vi "arraytest.vi"() -> ()   [LabVIEW 2010]
panel:
  out "Array 4":i32[][](array[numeric])
  out "Array 3":i32[](array[numeric])
  out "Array 2":bool[](array[boolean])
  out "Array":bool[][](array[boolean])
  out "x+y 2":dbl
  in  "Stopp 2":bool
  out "zeit":dbl
  out "Teil-Array":dbl[](array[numeric])
  in  "Index (Zeile)":i32
  in  "Zykluslänge [s]":i32
  out "XY-Graph":cluster{dbl[], dbl[]}[](graph)
  out "Boolesch 2":bool=TRUE
  out "Boolesch":bool=TRUE
  in  "Stopp":bool
  out "x+y":dbl[](array[numeric])
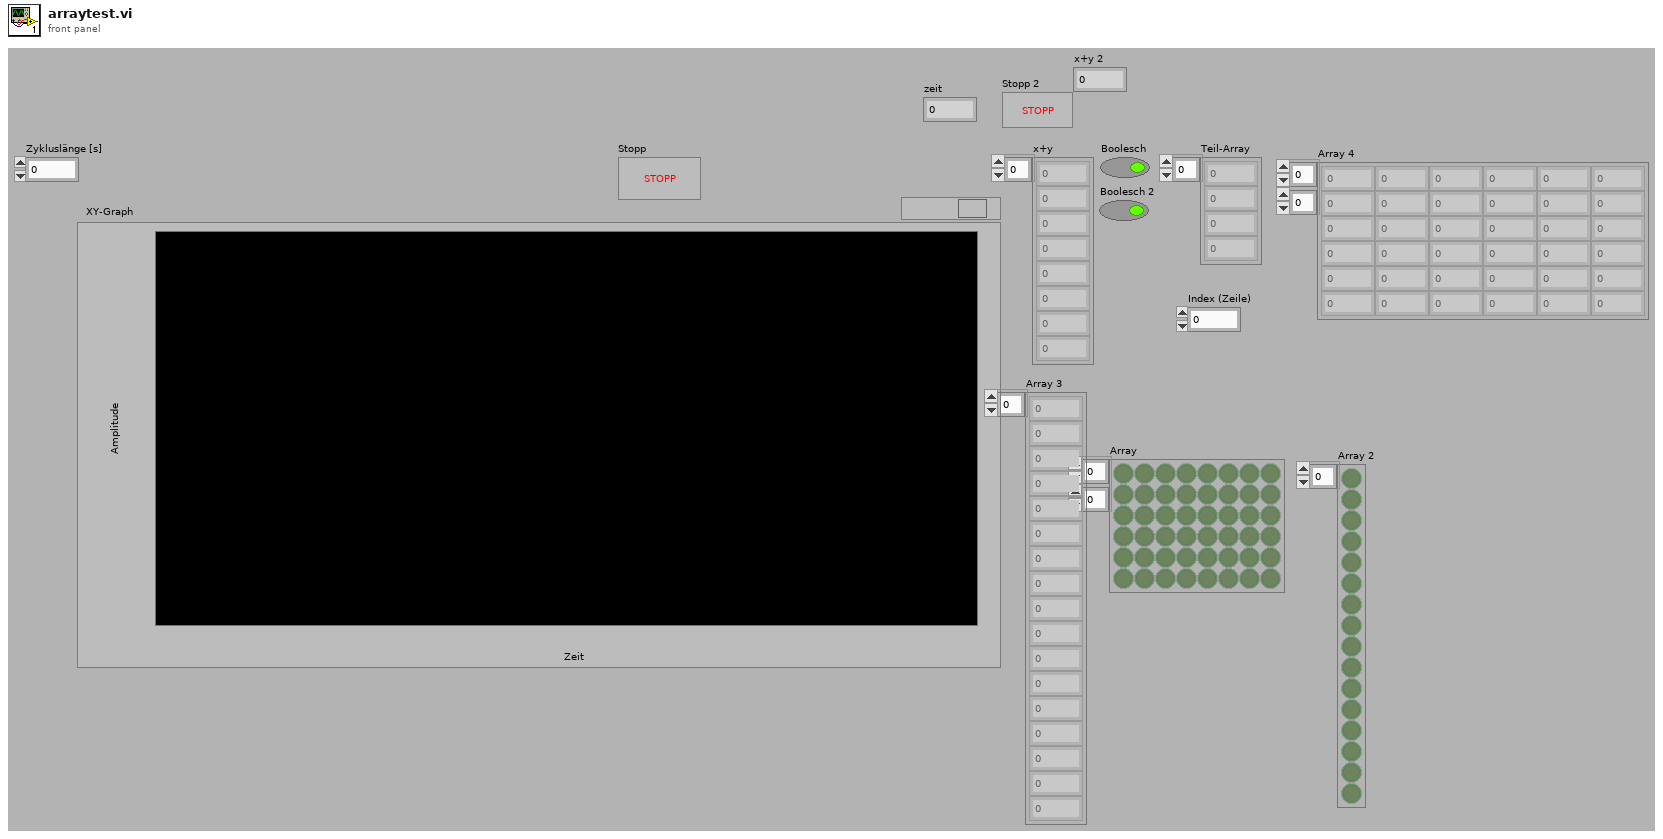
[diagram p1: front panel]
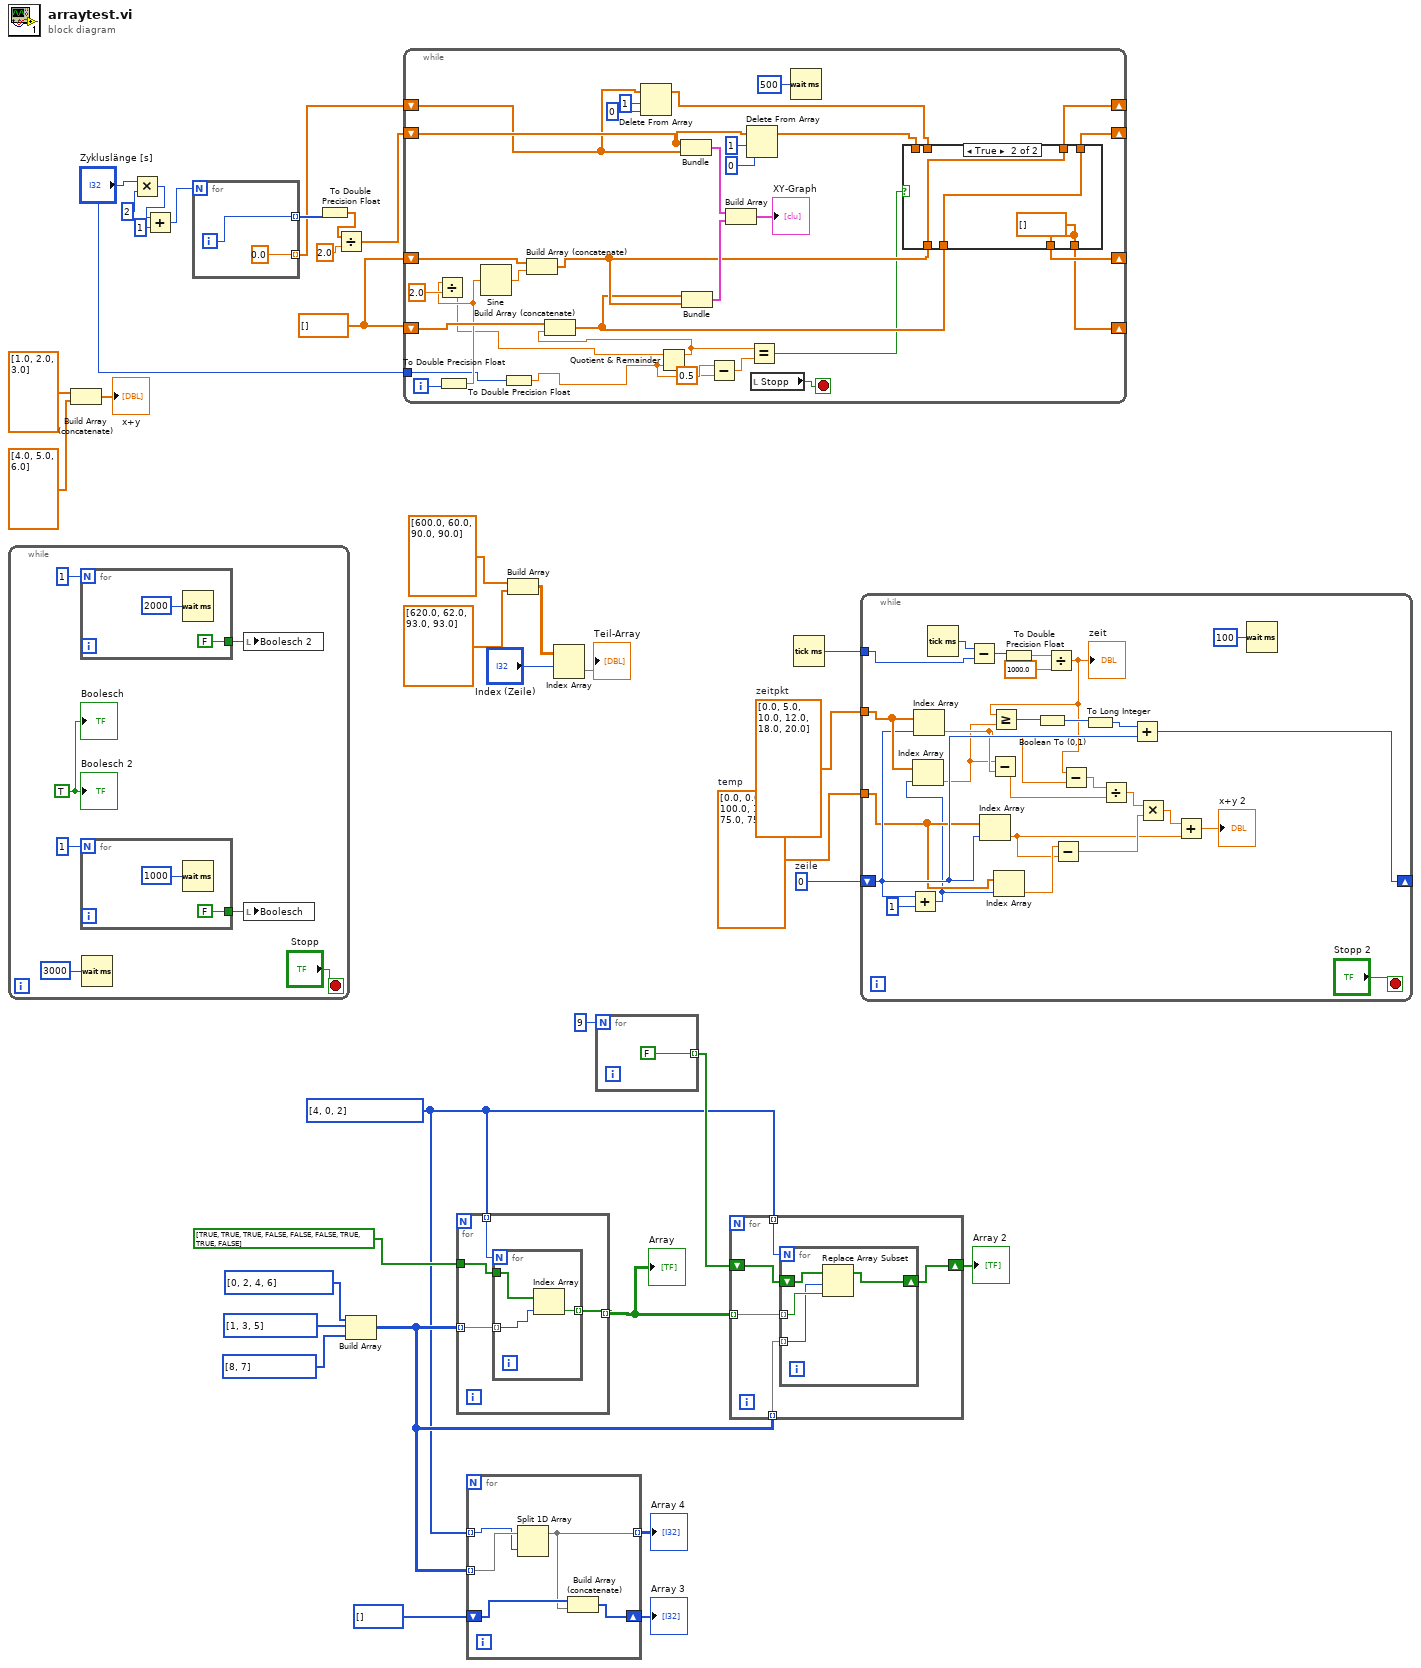
[diagram p0: block diagram]
diagram:
  w4 = i32[] [4, 0, 2]
  w14 = 0  # zeile
  w15 = dbl[] [0.0, 0.0, 100.0, 100.0, 75.0, 75.0]  # temp
  w16 = dbl[] [0.0, 5.0, 10.0, 12.0, 18.0, 20.0]  # zeitpkt
  w24 = dbl[] []
  n1 = while {
    stop <- "Stopp" stop-if-true
    w42 = TRUE ("Boolesch")
    n2 = for {
      N: 1 -> [_]
      tunnel: [FALSE] -> w39
      n3 = Wait (ms)(milliseconds to wait=u32 2000 ("Zu wartende ms")) -> ()  [unwired: 1 out]
    }
    n4 = for {
      N: 1 -> [_]
      tunnel: [FALSE] -> w40
      n5 = Wait (ms)(milliseconds to wait=u32 1000 ("Zu wartende ms")) -> ()  [unwired: 1 out]
    }
    n6 = Wait (ms)(milliseconds to wait=u32 3000 ("Zu wartende ms")) -> ()  [unwired: 1 out]
    n7 = local write "Boolesch 2"(w39) -> ()
    n8 = local write "Boolesch"(w40) -> ()
    "Boolesch" <- w42
    "Boolesch 2" <- w42
  }
  n9 = Build Array (concatenate)(dbl[] [1.0, 2.0, 3.0], dbl[] [4.0, 5.0, 6.0]) -> (→"x+y":dbl[])
  n10 = Multiply(x="Zykluslänge [s]", y=2) -> (x*y=w32:i32)
  n11 = Add(x=w32, y=1) -> (x+y=w30:i32)
  n12 = for {
    N: w30 -> [_]
    tunnel: [w48] -> w29 mode=indexing
    tunnel: [0.0] -> w25 mode=indexing
    i -> [w48]
  }
  n13 = To Double Precision Float(number=w29) -> (double precision float=w28:dbl[])
  n14 = Divide(x=w28, y=2.0) -> (x/y=w26:dbl[])
  n15 = Build Array(i32[] [0, 2, 4, 6], i32[] [1, 3, 5], i32[] [8, 7]) -> (w5:i32[][])
  n16 = while {
    shift-right: [w62] -> _
    shift-left: w26 -> [w76]
    shift-right: [w64] -> _
    shift-left: w25 -> [w73]
    shift-right: [w58] -> _
    shift-left: w24 -> [w70]
    shift-right: [w60] -> _
    shift-left: w24 -> [w68]
    tunnel: "Zykluslänge [s]" -> [w56]
    i -> [w57]
    stop <- w81 stop-if-true
    n17 = To Double Precision Float(number=w57) -> (double precision float=w66:dbl)
    n18 = Divide(x=w66, y=2.0) -> (x/y=w55:dbl)
    n19 = Sine(x=w66) -> (sin(x)=w67:dbl)
    n20 = To Double Precision Float(number=w56) -> (double precision float=w53:dbl)
    n21 = Build Array (concatenate)(w68, w67) -> (w61:dbl[])
    n22 = Delete From Array(array=w73, length=1 ("Länge"), index=0 ("Index")) -> (array with subset deleted=w65:dbl[])  [unwired: 1 out]
    n23 = Quotient & Remainder(x=w55, y=w53) -> (x-y*floor(x/y)=w54:dbl)  [unwired: 1 out]
    n24 = Build Array (concatenate)(w70, w54) -> (w59:dbl[])
    n25 = Bundle(w76, w73) -> (w80:cluster{dbl[], dbl[]})  [unwired: 1 in]
    n26 = Bundle(w59, w61) -> (w79:cluster{dbl[], dbl[]})  [unwired: 1 in]
    n27 = Subtract(x=w53, y=0.5) -> (x-y=w51:dbl)
    n28 = Build Array(w80, w79) -> (→"XY-Graph":cluster{dbl[], dbl[]}[])
    n29 = Delete From Array(array=w76, length=1 ("Länge"), index=0 ("Index")) -> (array with subset deleted=w63:dbl[])  [unwired: 1 out]
    n30 = Equal?(x=w54, y=w51) -> (x = y?=w50:bool)
    n31 = local read "Stopp"() -> (w81:bool)
    n32 = Wait (ms)(milliseconds to wait=u32 500 ("Zu wartende ms")) -> ()  [unwired: 1 out]
    n33 = case shown="True" w50 {
      tunnel: w65 -> [w85 _]
      tunnel: [w85 w86] -> w64
      tunnel: w63 -> [w84 _]
      tunnel: [w84 w87] -> w62
      tunnel: w61 -> [w83 w86]
      tunnel: [w83 w88] -> w60
      tunnel: w59 -> [w82 w87]
      tunnel: [w82 w88] -> w58
      frame False {
      }
      frame True {
        w88 = dbl[] []
      }
    }
  }
  n34 = for {
    tunnel: bool[] [TRUE, TRUE, TRUE, FALSE, FALSE, FALSE, TRUE, TRUE, FALSE] -> [w92]
    tunnel: w5 -> [w91] mode=indexing
    tunnel: [w90] -> w7 mode=indexing
    tunnel: w4 -> [w89] mode=indexing
    n35 = for {
      N: w89 -> [_]
      tunnel: w92 -> [w95]
      tunnel: w91 -> [w94] mode=indexing
      tunnel: [w93] -> w90 mode=indexing
      n36 = Index Array(array=w95, index=w94) -> (element=w93:bool)
    }
  }
  "Array" <- w7
  n37 = for {
    tunnel: w5 -> [w98] mode=indexing
    tunnel: w4 -> [w97] mode=indexing
    shift-right: [w99] -> w2
    shift-left: i32[] [] -> [w100]
    tunnel: [w96] -> w1 mode=indexing
    n38 = Split 1D Array(array=w98, index=w97) -> (first subarray=w96:i32[])  [unwired: 1 out]
    n39 = Build Array (concatenate)(w100, w96) -> (w99:i32[])
  }
  "Array 3" <- w2
  "Array 4" <- w1
  n40 = Build Array(dbl[] [600.0, 60.0, 90.0, 90.0], dbl[] [620.0, 62.0, 93.0, 93.0]) -> (w20:dbl[][])
  n41 = Index Array(array=w20, index (row)="Index (Zeile)") -> (element=→"Teil-Array":dbl[])  [unwired: 1 in]
  n42 = for {
    N: 9 -> [_]
    tunnel: [FALSE] -> w8 mode=indexing
  }
  n43 = for {
    tunnel: w7 -> [w104] mode=indexing
    shift-right: [w105] -> w6
    shift-left: w8 -> [w106]
    tunnel: w4 -> [w103] mode=indexing
    tunnel: w5 -> [w102] mode=indexing
    n44 = for {
      N: w103 -> [_]
      shift-right: [w107] -> w105
      shift-left: w106 -> [w110]
      tunnel: w104 -> [w109] mode=indexing
      tunnel: w102 -> [w108] mode=indexing
      n45 = Replace Array Subset(array=w110, new element=w109, index=w108) -> (w107:bool[])
    }
  }
  "Array 2" <- w6
  n46 = Tick Count (ms)() -> (millisecond timer value=w17:u32)
  n47 = while {
    tunnel: w17 -> [w136]
    tunnel: w16 -> [w125]
    tunnel: w15 -> [w123]
    shift-right: [w127] -> _
    shift-left: w14 -> [w124]
    stop <- "Stopp 2" stop-if-true
    n48 = Add(x=w124, y=1) -> (x+y=w122:i32)
    n49 = Index Array(array=w125, index=w122) -> (element=w111:dbl)
    n50 = Index Array(array=w125, index=w124) -> (element=w119:dbl)
    n51 = Tick Count (ms)() -> (millisecond timer value=w137:u32)
    n52 = Subtract(x=w137, y=w136) -> (x-y=w135:u32)
    n53 = Index Array(array=w123, index=w124) -> (element=w113:dbl)
    n54 = Subtract(x=w111, y=w119) -> (x-y=w117:dbl)
    n55 = Index Array(array=w123, index=w122) -> (element=w121:dbl)
    n56 = To Double Precision Float(number=w135) -> (double precision float=w134:dbl)
    n57 = Divide(x=w134, y=1000.0) -> (x/y=w120:dbl)
    "zeit" <- w120
    n58 = Greater Or Equal?(x=w120, y=w111) -> (x >= y?=w130:bool)
    n59 = Boolean To (0,1)(Boolean=w130) -> (0, 1=w129:i16)
    n60 = Subtract(x=w121, y=w113) -> (x-y=w115:dbl)
    n61 = Subtract(x=w120, y=w119) -> (x-y=w118:dbl)
    n62 = To Long Integer(number=w129) -> (32bit integer=w128:i32)
    n63 = Divide(x=w118, y=w117) -> (x/y=w116:dbl)
    n64 = Add(x=w128, y=w124) -> (x+y=w127:i32)
    n65 = Multiply(x=w116, y=w115) -> (x*y=w114:dbl)
    n66 = Add(x=w114, y=w113) -> (x+y=→"x+y 2":dbl)
    n67 = Wait (ms)(milliseconds to wait=u32 100 ("Zu wartende ms")) -> ()  [unwired: 1 out]
  }
